vi "Create Device Tree.vi"(10 "Device Tree Items":T1(array[cluster]) caption="设备树项目", 11 "Device Tree Ref":refnum<vi> caption="设备树引用") -> ()   [LabVIEW 2015]
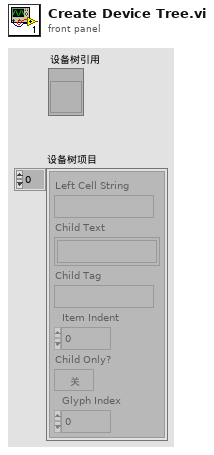
[diagram p1: front panel]
types:
  T1 = cluster{"Left Cell String":string, "Child Text":string[], "Child Tag":string, "Item Indent":i32, "Child Only?":bool, "Glyph Index":i32}[]
  T2 = cluster{"image type":i32, "image depth":i32, "image":u8[], "mask":u8[], "colors":u32[], "Rectangle":cluster{"left":i16, "top":i16, "right":i16, "bottom":i16}}[]
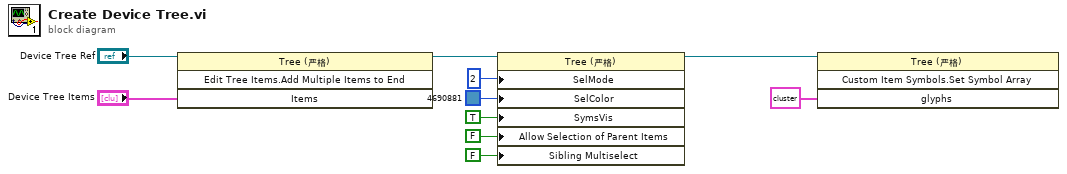
[diagram p0: block diagram]
diagram:
  n1 = invoke class="Tree (严格)" method="Edit Tree Items.Add Multiple Items to End"(reference="Device Tree Ref", "Items"="Device Tree Items") -> (reference out=w10:refnum<vi>)  [unwired: 2 in, 3 out]
  n2 = property class="Tree (严格)"(reference=w10, "SelMode"=2 ("选择模式"), "SelColor"=u32 4690881, "SymsVis"=TRUE ("显示项:显示符号"), "Allow Selection of Parent Items"=FALSE ("允许选择父项"), "Sibling Multiselect"=FALSE ("同辈多选")) -> (reference out=w7:refnum<vi>)  [unwired: 1 in, 1 out]
  n3 = invoke class="Tree (严格)" method="Custom Item Symbols.Set Symbol Array"(reference=w7, "glyphs"=T2 [{"image type"=0, "image depth"=0, "image"=[], "mask"=[], "colors"=[], "Rectangle"={"left"=0, "top"=0, "right"=0, "bottom"=0}}, {"image type"=0, "image depth"=32, "image"=array[1024 elements], "mask"=[0, 0, 63, 255, 127, 255, 127, 255, 127, 254, 127, 254, 127, 255, 127, 255, 127, 255, 127, 255, 127, 255, 127, 254, 127, 254, 127, 255, 127, 255, 63, 255], "colors"=[], "Rectangle"={"left"=0, "top"=0, "right"=16, "bottom"=16}}, {"image type"=0, "image depth"=32, "image"=array[1024 elements], "mask"=[0, 1, 127, 255, 255, 255, 255, 255, 255, 255, 255, 255, 255, 255, 255, 255, 255, 255, 255, 255, 255, 255, 255, 255, 255, 255, 255, 255, 127, 255, 7, 252], "colors"=[], "Rectangle"={"left"=0, "top"=0, "right"=16, "bottom"=16}}, {"image type"=0, "image depth"=32, "image"=array[1024 elements], "mask"=[0, 48, 127, 248, 127, 252, 255, 255, 255, 255, 255, 255, 255, 255, 127, 255, 127, 255, 127, 255, 127, 255, 127, 252, 127, 248, 127, 248, 127, 248, 0, 120], "colors"=[], "Rectangle"={"left"=0, "top"=0, "right"=16, "bottom"=16}}, {"image type"=0, "image depth"=32, "image"=array[1024 elements], "mask"=[0, 0, 66, 16, 103, 56, 61, 238, 16, 132, 0, 0, 93, 220, 85, 84, 119, 118, 0, 0, 3, 128, 3, 128, 3, 128, 31, 240, 15, 224, 30, 240], "colors"=[], "Rectangle"={"left"=0, "top"=0, "right"=16, "bottom"=16}}, {"image type"=0, "image depth"=32, "image"=array[1024 elements], "mask"=[0, 48, 127, 248, 127, 252, 255, 255, 255, 255, 255, 255, 255, 255, 127, 255, 127, 255, 127, 255, 127, 255, 127, 252, 127, 248, 127, 248, 127, 248, 0, 120], "colors"=[], "Rectangle"={"left"=0, "top"=0, "right"=16, "bottom"=16}}, {"image type"=0, "image depth"=32, "image"=array[1024 elements], "mask"=[0, 0, 66, 16, 103, 56, 61, 238, 16, 132, 0, 0, 93, 220, 85, 84, 119, 118, 0, 0, 3, 128, 3, 128, 3, 128, 31, 240, 15, 224, 30, 240], "colors"=[], "Rectangle"={"left"=0, "top"=0, "right"=16, "bottom"=16}}] ("自定义项符号:获取符号数组")) -> ()  [unwired: 2 in, 4 out]
